vi "zeroes_1d.vi"(2 "m":i32=1) -> (7 "ones":dbl[](array[numeric]))   [LabVIEW 2018, in "NI_Gmath.lvlib"]
uses:
  NI_Gmath.lvlib
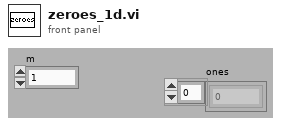
[diagram p1: front panel]
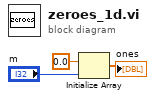
[diagram p0: block diagram]
diagram:
  n1 = Initialize Array(0.0 ("element"), "m") -> (→"ones":dbl[])
